vi "Robot Main.vi"() -> ()   [LabVIEW 2023]
doc: "This VI implements the framework and scheduler for your robotics program. It should not be necessary to modify the framework. You are expected to add your code to the VIs called from Robot Main - the ones located in the Team Code folder within the project."
uses:
  <vilib>/Rock Robotics/WPI/Camera/WPI_CameraImageSize.ctl
  Robot Global Data.vi
panel:
  out "agitator sweeps/s":dbl=1.0 step=0.1
  out "Score":dbl
  out "Distance":dbl
  out "scoop speed":dbl=0.7 step=0.1
  out "shooter speed":dbl=0.85 min=-1.0 max=1.0 step=0.01
  in  "Image Size":T1=enum."320x240"
  in  "Enable Vision":bool
  in  "Finish":bool
  # "This robot project is intended for learning LabVIEW for FRC, and running a predefined robot in a simulated environment.  You should run this Robot Main.vi in debug mode (press the Run arrow).  For more information on programing the simulated robot, open the Robot Simulation Readme.html file in the project.\n\nThis robot project has a matching dashboard project:\nDashboard for Ball Shooter Robot\nCreate that project from the dashboard wizard and run Dashboard Main.vi. It will allow you to control the shooter motors, scoop motors, and agitator motor. It also shows orientation, distance to the wall, and scoring.\n\nThe dashboard wizard can be found by choosing:\nView>>Getting Started Window...\nand then clicking FRC Dashboard Project\n\nIf you already have a Dashboard exe running, you should close it before running this new one."
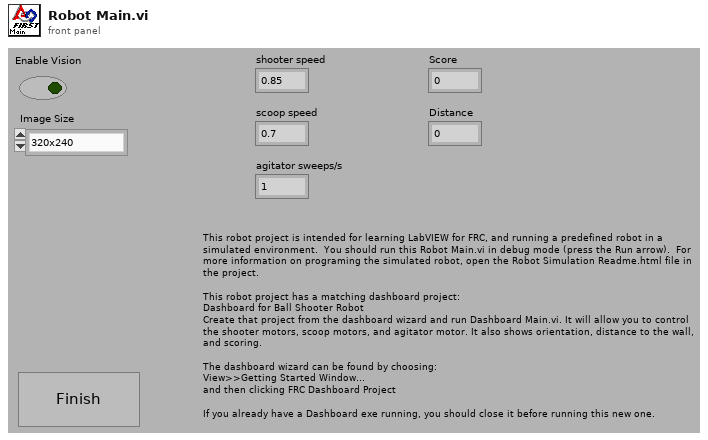
[diagram p1: front panel]
types:
  T1 = typedef "WPI_CameraImageSize.ctl" = enum16{"640x480", "320x240", "160x120", "Custom"}
  T2 = typedef "WPI_DriverStationMatch Info.ctl" = cluster{"Autonomous Elapsed Seconds":dbl, "TeleOp Elapsed Seconds":dbl, "Disabled Elapsed Seconds":dbl, "Visited Autonomous":bool, "Visited TeleOp":bool, "Visited Disabled":bool, "Autonomous Settings":cluster{"Autonomous Style":enum16{"Iterative", "Independent"}, "VI Refnum":refnum<vi>}}
  T3 = typedef "WPI_DriverStationDerivedRobotMode.ctl" = enum16{"Init", "Execute", "Stop"}
  T4 = typedef "WPI_DriverStationRobotMode2.ctl" = enum16{"Autonomous Disabled", "Autonomous Enabled", "Teleop Disabled", "Teleop Enabled", "Disconnected", "Finish", "Test Disabled", "Test Enabled", "Emergency Stopped"}
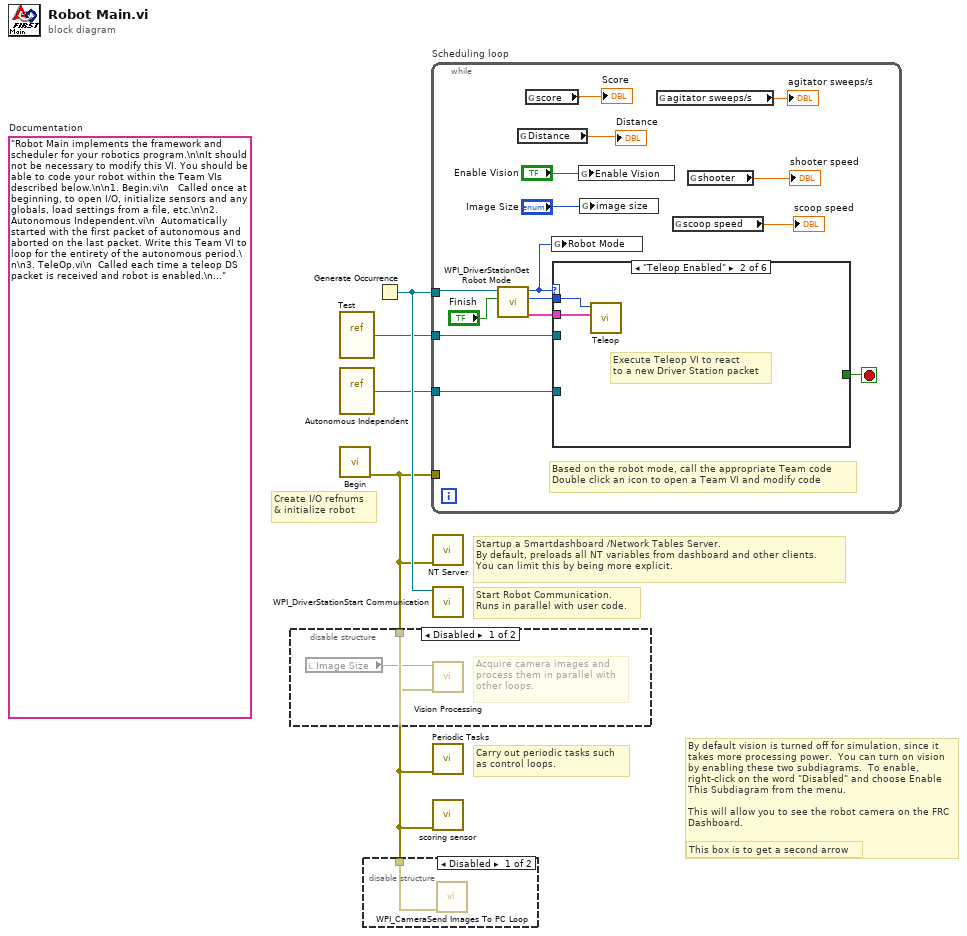
[diagram p0: block diagram]
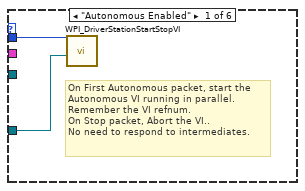
[diagram p4: hidden frame]
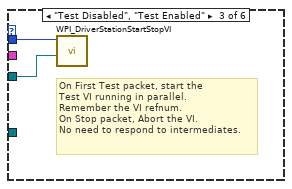
[diagram p5: hidden frame]
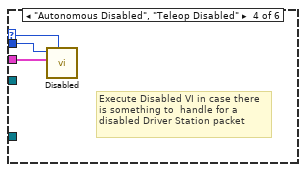
[diagram p6: hidden frame]
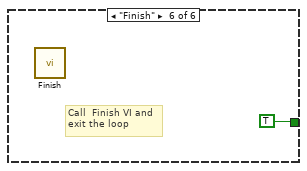
[diagram p8: hidden frame]
diagram:
  (unwired) "Robot Main implements the framework and scheduler for your robotics program.\n\nIt should not be necessary to modify this VI. You should be able to code your robot within the Team VIs described below.\n\n1. Begin.vi\n   Called once at beginning, to open I/O, initialize sensors and any globals, load settings from a file, etc.\n\n2. Autonomous Independent.vi\n  Automatically started with the first packet of autonomous and aborted on the last packet. Write this Team VI to loop for the entirety of the autonomous period.\n\n3. TeleOp.vi\n  Called each time a teleop DS packet is received and robot is enabled.\n\n4. Disabled.vi\n  Called each time a packet is received and the robot is disabled.\n\n5. Test.vi\n  Called Automatically started with the first test packet and aborted on the last. Modify this VI to carry out robot and sensor validation tests.\n\n6. Vision.vi\n  A parallel loop that acquires and processes camera images.\n\n7. PeriodicTasks.vi\n  Parallel loops running at user-defined rates.\n\n8. Finish.vi\n  Called before exiting, so you can save data, clean up I/O, etc.\n"  # Documentation
  # "By default vision is turned off for simulation, since it takes more processing power.  You can turn on vision by enabling these two subdiagrams.  To enable, right-click on the word \"Disabled\" and choose Enable This Subdiagram from the menu.\n\nThis will allow you to see the robot camera on the FRC Dashboard."
  # "Startup a Smartdashboard /Network Tables Server.\nBy default, preloads all NT variables from dashboard and other clients.\nYou can limit this by being more explicit."
  # "Carry out periodic tasks such\nas control loops."
  # "Create I/O refnums\n& initialize robot"
  # "Start Robot Communication.\nRuns in parallel with user code."
  # "This box is to get a second arrow"
  n1 = vi-ref "Test.vi"() -> (w2:refnum<vi>)
  n2 = vi-ref "Autonomous Independent.vi"() -> (w3:refnum<vi>)
  n3 = call "Begin.vi"() -> ("error out"=w1:errorcluster)  [unwired: 2 in, 9 out]
  n4 = disable-structure shown="Disabled" {
    disable-tunnel: w1 -> [w5 _]
    frame Disabled {
      # "Acquire camera images and\nprocess them in parallel with\nother loops."
      n5 = local read "Image Size"() -> (w6:T1)
      n6 = call "Vision Processing.vi"("error in (no error)"=w5, "Image Size"=w6) -> ()  [unwired: 6 out]
    }
    frame Enabled {
    }
  }
  n7 = disable-structure shown="Disabled" {
    disable-tunnel: w1 -> [w7 _]
    frame Disabled {
      n8 = call <vilib>:"WPI_CameraSend Images To PC Loop.vi"("error in (no error)"=w7) -> ()  [unwired: 11 in]
    }
    frame Enabled {
    }
  }
  n9 = Generate Occurrence() -> (w4:refnum<k4>)
  n10 = while "Scheduling loop" {
    tunnel: w4 -> [w21]
    tunnel: w1 -> [_]
    tunnel: w3 -> [w16]
    tunnel: w2 -> [w14]
    stop <- w18 stop-if-true
    # "Based on the robot mode, call the appropriate Team code\nDouble click an icon to open a Team VI and modify code"
    n11 = call <vilib>:"WPI_DriverStationGet Robot Mode.vi"("Finish"="Finish", "DS Occurrence"=w21) -> ("Match Info out"=w19:T2, "Call Context"=w22:T3, "Robot Mode"=w13:T4)  [unwired: 7 out]
    n12 = global read "Robot Global Data.vi" "Distance"() -> (→"Distance":dbl)
    n13 = global read "Robot Global Data.vi" "score"() -> (→"Score":dbl)
    n14 = global write "Robot Global Data.vi" "Robot Mode"(w13) -> ()
    n15 = case shown="\"Teleop Enabled\"" w13 {
      selector: w13 -> [_ _ _ w29 _ _]
      tunnel: w22 -> [w24 w26 w28 w31 _ _]
      tunnel: w19 -> [_ w25 _ w30 _ _]
      tunnel: [_ _ _ _ _ TRUE] -> w18
      tunnel: w16 -> [w23 _ _ _ _ _]
      tunnel: w14 -> [_ _ w27 _ _ _]
      frame "Autonomous Enabled" {
        # "On First Autonomous packet, start the\nAutonomous VI running in parallel.\nRemember the VI refnum.\nOn Stop packet, Abort the VI..\nNo need to respond to intermediates."
        n16 = call <vilib>:"WPI_DriverStationStartStopVI.vi"("VI in"=w23, "Call Context"=w24) -> ()  [unwired: 10 in]
      }
      frame "Teleop Enabled" {
        # "Execute Teleop VI to react\nto a new Driver Station packet"
        n17 = call "Teleop.vi"("Match Info"=w25, "Call Context"=w26) -> ()  [unwired: 1 in, 9 out]
      }
      frame "Test Disabled", "Test Enabled" {
        # "On First Test packet, start the\nTest VI running in parallel.\nRemember the VI refnum.\nOn Stop packet, Abort the VI.\nNo need to respond to intermediates."
        n18 = call <vilib>:"WPI_DriverStationStartStopVI.vi"("VI in"=w27, "Call Context"=w28) -> ()  [unwired: 10 in]
      }
      frame "Autonomous Disabled", "Teleop Disabled" {
        # "Execute Disabled VI in case there\nis something to  handle for a\ndisabled Driver Station packet"
        n19 = call "Disabled.vi"("Robot Mode"=w29, "Match Info"=w30, "Call Context"=w31) -> ()  [unwired: 1 in, 8 out]
      }
      frame "Disconnected", Default {
        # "Driver Station packet didn't arrive.\nPossibly useful for diagnostics"
      }
      frame "Finish" {
        # "Call  Finish VI and\nexit the loop"
        n20 = call "Finish.vi"() -> ()  [unwired: 1 in, 7 out]
      }
    }
    n21 = global write "Robot Global Data.vi" "Enable Vision"("Enable Vision") -> ()
    n22 = global write "Robot Global Data.vi" "image size"("Image Size") -> ()
    n23 = global read "Robot Global Data.vi" "agitator sweeps/s"() -> (→"agitator sweeps/s":dbl)
    n24 = global read "Robot Global Data.vi" "scoop speed"() -> (→"scoop speed":dbl)
    n25 = global read "Robot Global Data.vi" "shooter"() -> (→"shooter speed":dbl)
  }
  n26 = call <vilib>:"NT Server.vi"("error in (no error)"=w1) -> ()  [unwired: 10 in, 1 out]
  n27 = call <vilib>:"WPI_DriverStationStart Communication.vi"("occurrence"=w4) -> ()  [unwired: 2 in, 9 out]
  n28 = call "Periodic Tasks.vi"("error in"=w1) -> ()  [unwired: 1 in, 10 out]
  n29 = call "scoring sensor.vi"("error in"=w1) -> ()  [unwired: 11 in]
